vi "B_1.vi"() -> ()   [LabVIEW 2020]
uses:
  <vilib>/numeric/Random Number (Range) I64.vi
  <vilib>/numeric/sub_Random U32.vi
panel:
  out "Number":i64[](array[numeric])
  out "Even numb":i64[](array[numeric])
  out "Odd numb":i64[](array[numeric])
  in  "Amout of numb":i32
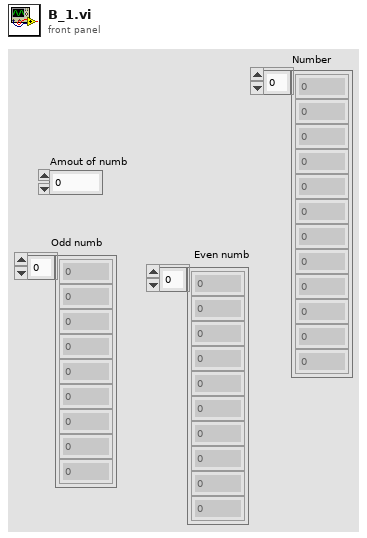
[diagram p1: front panel]
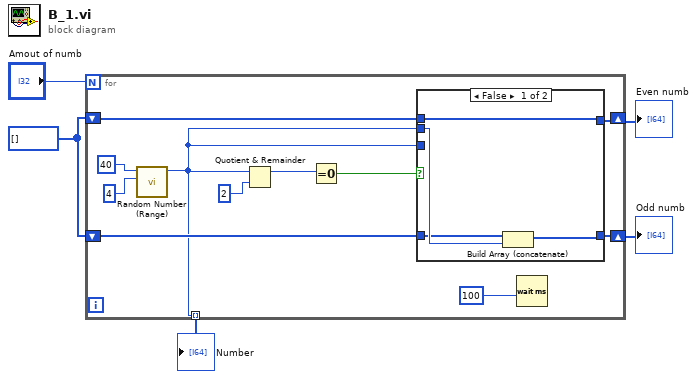
[diagram p0: block diagram]
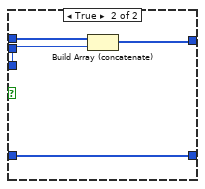
[diagram p2: hidden frame]
diagram:
  w1 = i64[] [] ("Array")
  n1 = for {
    N: "Amout of numb" -> [_]
    shift-right: [w14] -> w5
    shift-left: w1 -> [w15]
    shift-right: [w12] -> w4
    shift-left: w1 -> [w13]
    tunnel: [w8] -> w3 mode=indexing
    n2 = call-poly <vilib>:"Random Number (Range).vi"("lower bound (-100)"=i64 4, "upper bound (100)"=i64 40) -> ("number"=w8:i64)  [unwired: 9 in]
    n3 = Quotient & Remainder(x=w8, y=i64 2 ("floor(x/y)")) -> (x-y*floor(x/y)=w7:i64)  [unwired: 1 out]
    n4 = Equal To 0?(x=w7) -> (x = 0?=w6:bool)
    n5 = case shown="False" w6 {
      tunnel: w8 -> [_ w24]
      tunnel: w15 -> [w17 w23]
      tunnel: [w17 w22] -> w14
      tunnel: w13 -> [w19 w21]
      tunnel: [w18 w21] -> w12
      tunnel: w8 -> [w20 _]
      frame False {
        n6 = Build Array (concatenate)(w19, w20) -> (w18:i64[])
      }
      frame True {
        n7 = Build Array (concatenate)(w23, w24) -> (w22:i64[])
      }
    }
    n8 = Wait (ms)(milliseconds to wait=u32 100 ("millisecond timer value")) -> ()  [unwired: 1 out]
  }
  "Odd numb" <- w4
  "Even numb" <- w5
  "Number" <- w3
